vi "New Tag_From JSON Config.vi"(8 "error in (no error)":errorcluster, 10 "JSON Tag Config":string) -> (0 "error out":errorcluster, 2 "Tag Ref out":refnum<data-value>)   [LabVIEW 2020, in "Tag Engine.lvlib"]
doc: "Build a new Tag from a JSON config string.\n\nThe JSON config string must at least specify the Name, Type, Typestring, and initial value property."
uses:
  Tag Engine.lvlib
  Tag/Tag.lvclass
  Core/Tag Core.lvclass
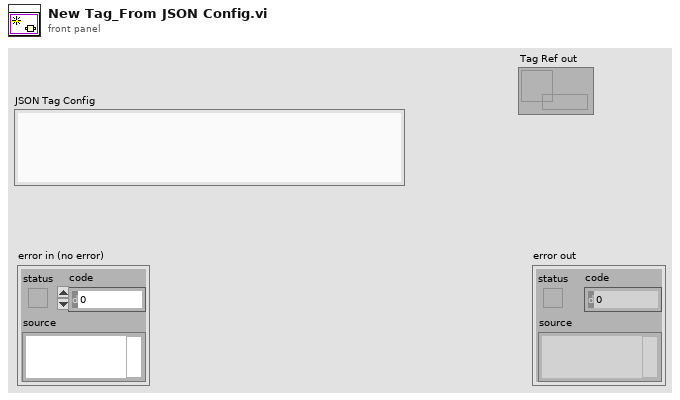
[diagram p1: front panel]
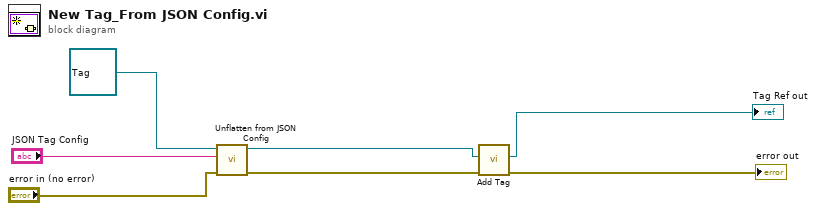
[diagram p0: block diagram]
diagram:
  n1 = call "Unflatten from JSON Config.vi"("error in (no error)"="error in (no error)", "JSON Text"="JSON Tag Config", "Tag in"=refnum<class "Tag.lvclass"> refnum ("CVT Item in")) -> ("error out"=w3:errorcluster, "Tag out"=w2:refnum<class "Tag.lvclass">)  [unwired: 7 in]
  n2 = call "Add Tag.vi"("error in (no error)"=w3, "Tag in"=w2) -> ("error out"=→"error out":errorcluster, "Tag Reference out"=→"Tag Ref out":refnum<data-value>)  [unwired: 8 in]
